vi "gxml_BlindArraySize.vi"(7 "Current Array Info":cluster{"Hierarchy":string, "Item Name":string}, 8 "error in":errorcluster, 9 "Encaps Array Info":T1, 11 "Dim Attr":string) -> (0 "error out":errorcluster, 1 "Encaps Array Info":T1, 2 "Flattened Array Header":string, 3 "Number of Elements":i32)   [LabVIEW 2011, in "Third Party VIs.lvlib" / "GXML.lvlib"]
uses:
  <vilib>/regexp/Match Regular Expression.xnode
  GXML.lvlib
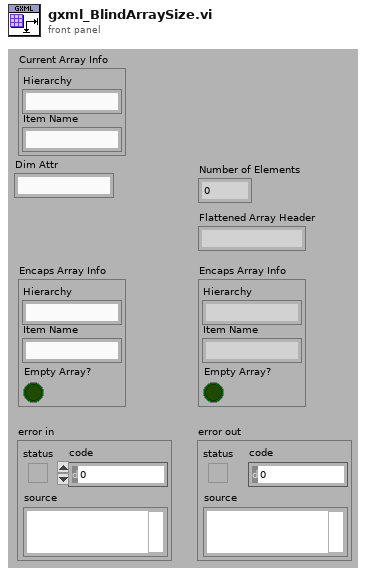
[diagram p1: front panel]
types:
  T1 = cluster{"Hierarchy":string, "Item Name":string, "Empty Array?":bool}
  T2 = cluster{"Hierarchy":string, "Item Name":string, bool}
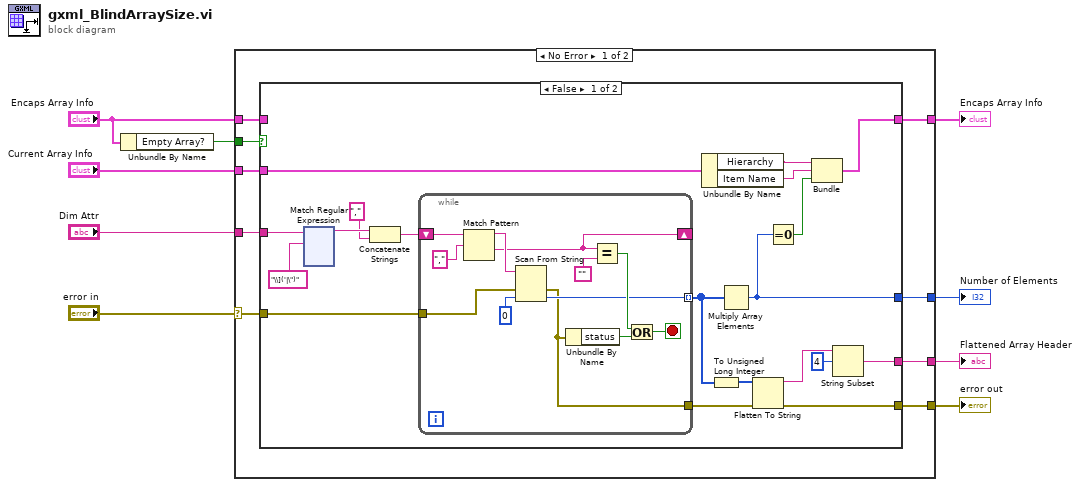
[diagram p0: block diagram]
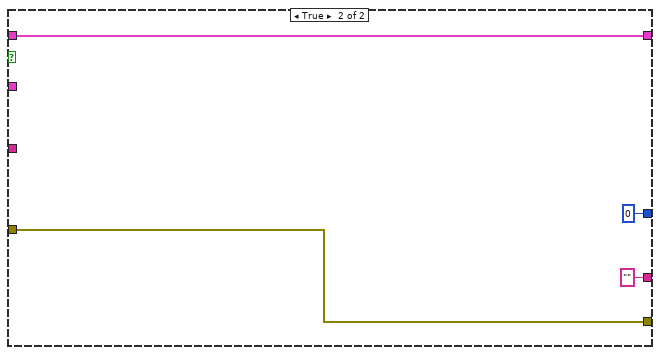
[diagram p2: hidden frame]
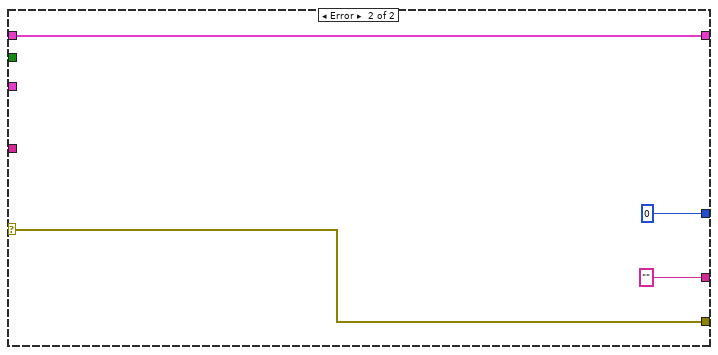
[diagram p3: hidden frame]
diagram:
  n1 = Unbundle By Name("Encaps Array Info") -> ("Empty Array?"=w1:bool)
  n2 = case shown="No Error" "error in" {
    selector: "error in" -> [w15 w166]
    tunnel: [w14 0] -> w9
    tunnel: "Dim Attr" -> [w18 _]
    tunnel: [w17 "" ("data string")] -> w7
    tunnel: [w16 w166] -> w6
    tunnel: [w10 w165] -> w4
    tunnel: "Current Array Info" -> [w11 _]
    tunnel: "Encaps Array Info" -> [w12 w165]
    tunnel: w1 -> [w13 _]
    frame No Error {
      n3 = case shown="False" w13 {
        tunnel: w18 -> [w19 _]
        tunnel: [w30 "" ("data string")] -> w17
        tunnel: [w27 w162] -> w16
        tunnel: w15 -> [w26 w162]
        tunnel: [w25 0] -> w14
        tunnel: w12 -> [_ w161]
        tunnel: w11 -> [w23 _]
        tunnel: [w20 w161] -> w10
        frame False {
          n4 = xnode "Match Regular Expression"("input string"=w19, "regular expression"="\\]('|\")") -> ("before match"=w36:string)  [unwired: 4 in, 4 out]
          n5 = Concatenate Strings(w36, ",") -> (w34:string)
          n6 = while {
            shift-right: [w156] -> _
            shift-left: w34 -> [w158]
            tunnel: [w151] -> w32 mode=indexing
            tunnel: [w150] -> w28
            tunnel: w26 -> [w149]
            stop <- w152 stop-if-true
            n7 = Match Pattern(string=w158, regular expression=",") -> (before substring=w157:string, after substring=w156:string)  [unwired: 1 in, 2 out]
            n8 = Scan From String(input string=w157, error in=w149, default 1=0) -> (error out=w150:errorcluster, output 1=w151:i32)  [unwired: 2 in, 2 out]
            n9 = Unbundle By Name(w150) -> ("status"=w154:bool)
            n10 = Equal?(x=w156, y="") -> (x = y?=w153:bool)
            n11 = Or(x=w153, y=w154) -> (x .or. y?=w152:bool)
          }
          n12 = Unbundle By Name(w23) -> ("Hierarchy"=w22:string, "Item Name"=w21:string)
          n13 = To Unsigned Long Integer(number=w32) -> (unsigned 32bit integer=w33:u32[])
          n14 = Multiply Array Elements(1:w32) -> (0:w25:i32)
          n15 = Flatten To String(anything=w33, error in (no error)=w28) -> (data string=w31:string, error out=w27:errorcluster)  [unwired: 2 in, 1 out]
          n16 = Equal To 0?(x=w25) -> (x = 0?=w24:bool)
          n17 = Bundle("Hierarchy"=w22, "Item Name"=w21, w24) -> (w20:T2)  [unwired: 1 in]
          n18 = String Subset(string=w31, offset (0)=4) -> (substring=w30:string)  [unwired: 1 in]
        }
        frame True {
        }
      }
    }
    frame Error {
    }
  }
  "Number of Elements" <- w9
  "Flattened Array Header" <- w7
  "error out" <- w6
  "Encaps Array Info" <- w4
